vi "create.vi"(8 "error in (no error)":errorcluster, 10 "Month":T1, 11 "YYYY":i32=2008) -> (0 "error out":errorcluster, 3 "WhichMonth out":refnum<class "WhichMonth.lvclass">)   [LabVIEW 2018, in "WhichMonth.lvclass"]
uses:
  WhichMonth.lvclass
  database/Month.ctl
  WhichMonth.lvclass/WhichMonth.ctl
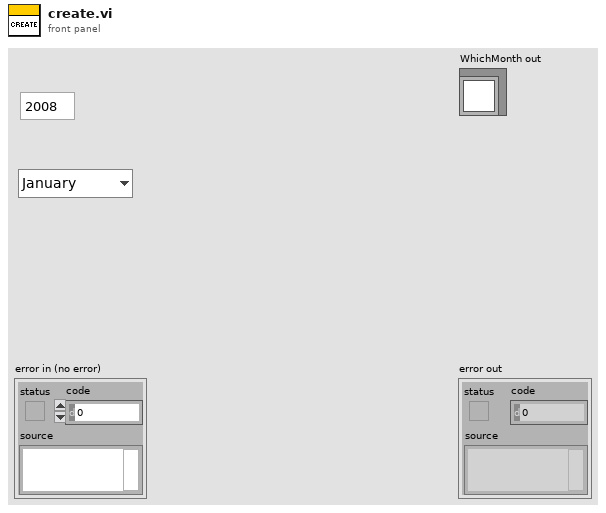
[diagram p1: front panel]
types:
  T1 = typedef "WhichMonth.lvclass/Month.ctl" = enum16{"January", "February", "March", "April", "May", "June", "July", "August", "September", "October", "November", "December"}
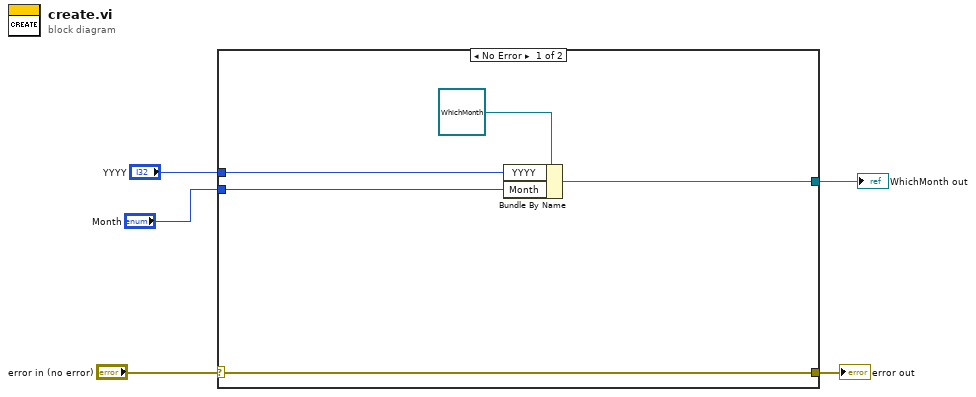
[diagram p0: block diagram]
diagram:
  n1 = case shown="No Error" "error in (no error)" {
    selector: "error in (no error)" -> [w10 w11]
    tunnel: [w10 w11] -> w4
    tunnel: "YYYY" -> [w8 _]
    tunnel: "Month" -> [w7 _]
    tunnel: [w6 _] -> w1
    frame No Error {
      n2 = Bundle By Name(cluster=refnum<class "WhichMonth.lvclass"> refnum ("WhichMonth in"), "YYYY"=w8, "Month"=w7) -> (w6:refnum<class "WhichMonth.lvclass">)
    }
    frame Error {
    }
  }
  "error out" <- w4
  "WhichMonth out" <- w1
